vi "main.vi"() -> ()   [LabVIEW 2014]
uses:
  <vilib>/Utility/error.llb/DialogType.ctl
panel:
  out "Sound graph of Combined":waveform(dbl)[](graph)
  out "Sound graph of 2":waveform(dbl)[](graph)
  out "Sound graph of 1":waveform(dbl)[](graph)
  out "error out":errorcluster
  in  "error in (no error)":errorcluster
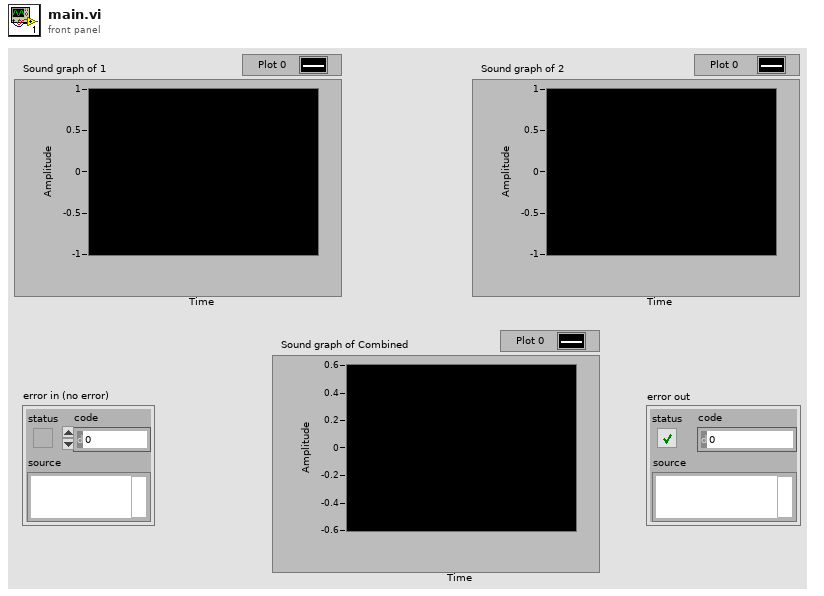
[diagram p1: front panel]
types:
  T1 = typedef "DialogType.ctl" = u16
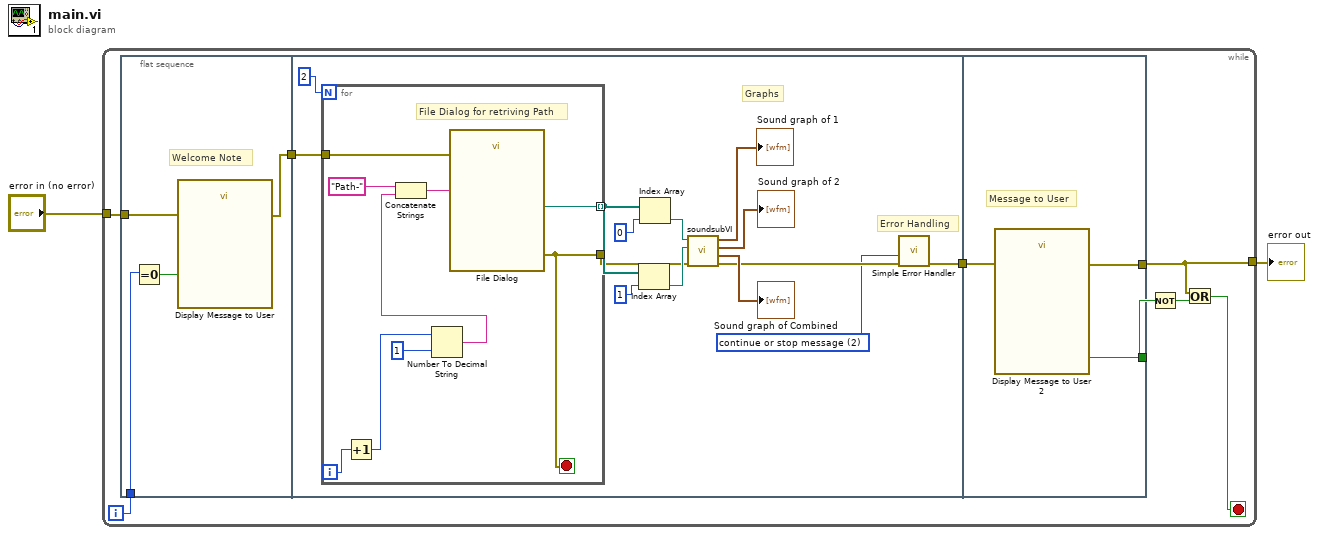
[diagram p0: block diagram]
diagram:
  n1 = while {
    tunnel: "error in (no error)" -> [w9]
    tunnel: [w4] -> w1
    i -> [w8]
    stop <- w5 stop-if-true
    n2 = flat-sequence {
      tunnel: w9 -> [w14]
      tunnel: [w13] -> w10
      tunnel: w8 -> [w11]
      tunnel: w10 -> [w19]
      tunnel: [w17] -> w3
      tunnel: [w40] -> w7
      tunnel: [w39] -> w4
      tunnel: w3 -> [w38]
      frame #0 {
        # "Welcome Note"
        n3 = Equal To 0?(x=w11) -> (x = 0?=w12:bool)
        n4 = call "Display Message to User"("error in (no error)"=w14, "Enable"=w12) -> ("error out"=w13:errorcluster)  [unwired: 8 in, 1 out]
      }
      frame #1 {
        w15 = T1 2 items=["no dialog", "OK message", "continue or stop message", "OK message + warnings", "continue/stop + warnings"] ("type of dialog (OK msg:1)")
        # "Error Handling"
        # "Graphs"
        n5 = for {
          N: 2 -> [_]
          tunnel: [w37] -> w24 mode=indexing
          tunnel: [w36] -> w18
          tunnel: w19 -> [w29]
          i -> [w31]
          stop <- w36 stop-if-true
          # "File Dialog for retriving Path"
          n6 = Increment(x=w31) -> (x+1=w30:i32)
          n7 = Number To Decimal String(number=w30, width (-)=i16 1) -> (decimal integer string=w33:string)
          n8 = Concatenate Strings("Path-" ("string"), w33) -> (w35:string)
          n9 = call "File Dialog"("prompt"=w35, "error in"=w29) -> ("selected path"=w37:path, "error out"=w36:errorcluster)  [unwired: 10 in, 2 out]
        }
        n10 = Index Array(array=w24, index=1) -> (element=w20:path)
        n11 = Index Array(array=w24, index=0) -> (element=w21:path)
        n12 = call "soundsubVI.vi"("error in (no error)"=w18, "Sound File 2"=w20, "Sound File 1"=w21) -> ("error out"=w16:errorcluster, "Sound graph of Combined"=→"Sound graph of Combined":waveform(dbl)[], "Sound graph of 2"=→"Sound graph of 2":waveform(dbl)[], "Sound graph of 1"=→"Sound graph of 1":waveform(dbl)[])  [unwired: 5 in]
        n13 = call <vilib>:"Simple Error Handler.vi"("type of dialog (OK msg:1)"=w15, "error in (no error)"=w16) -> ("error out"=w17:errorcluster)  [unwired: 3 in, 4 out]
      }
      frame #2 {
        # "Message to User"
        n14 = call "Display Message to User 2"("error in (no error)"=w38) -> ("error out"=w39:errorcluster, "OK"=w40:bool)  [unwired: 9 in]
      }
    }
    n15 = Not(x=w7) -> (.not. x?=w6:bool)
    n16 = Or(x=w4, y=w6) -> (x .or. y?=w5:bool)
  }
  "error out" <- w1
